vi "Test_SQLQueryVIM1DI64_WorksNoError.vi"(8 "error in (no error)":errorcluster, 11 "TestCase in":refnum<class "Test mysql.lvclass">) -> (0 "error out":errorcluster, 3 "TestCase out":refnum<class "Test mysql.lvclass">)   [LabVIEW 2020, in "DataBase_mysql_Tests.lvlib" / "Test mysql.lvclass"]
uses:
  Test mysql.lvclass
  98ffd0c8-4361-48ce-8721-6d705661544a.vi
  98ffd0c8-4361-48ce-8721-6d705661544a.vi/2b921c3d-a080-433c-a702-8a31cd1244f2.vi
  98ffd0c8-4361-48ce-8721-6d705661544a.vi/7350d3e2-eed7-4e35-bdb1-e124b5b41b91.vi
  <vilib>/Utility/error.llb/Error Cluster From Error Code.vi
  externals/mysql/Source/mysql.net/mysql.lvclass
  <vilib>/addons/_JKI Toolkits/VI Tester/TestCase.llb/TestCase.lvclass
  C:/Program Files/National Instruments/LabVIEW 2020/vi.lib/addons/_JKI Toolkits/VI Tester/TestCase.llb/TestCase.lvclass
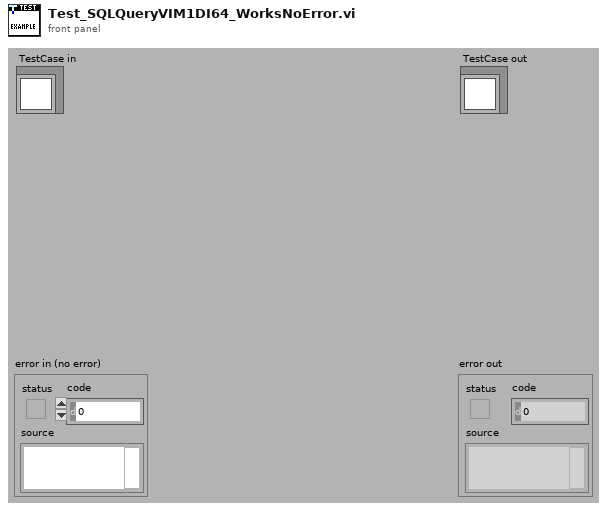
[diagram p1: front panel]
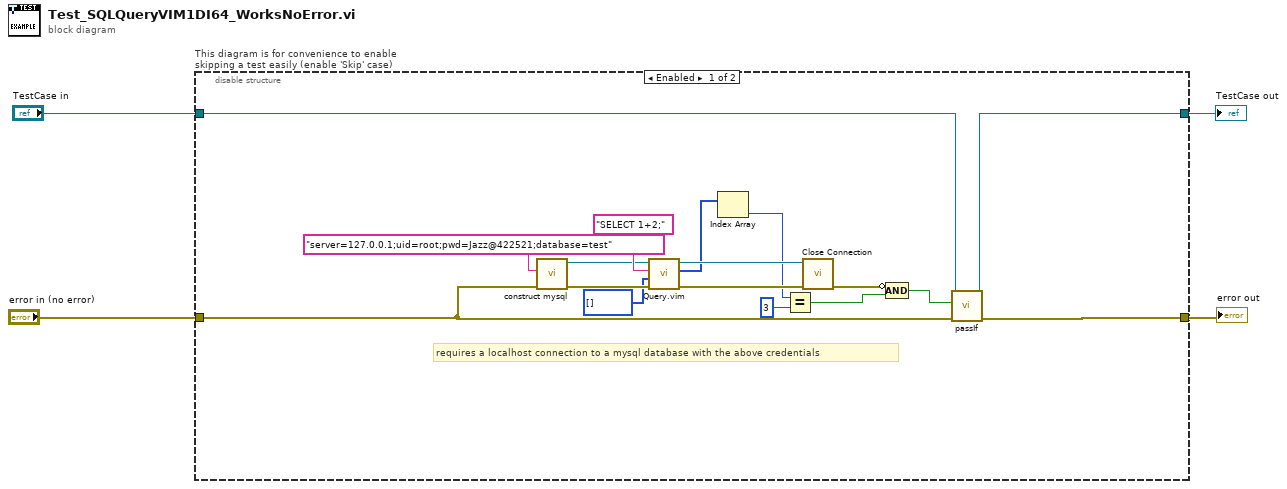
[diagram p0: block diagram]
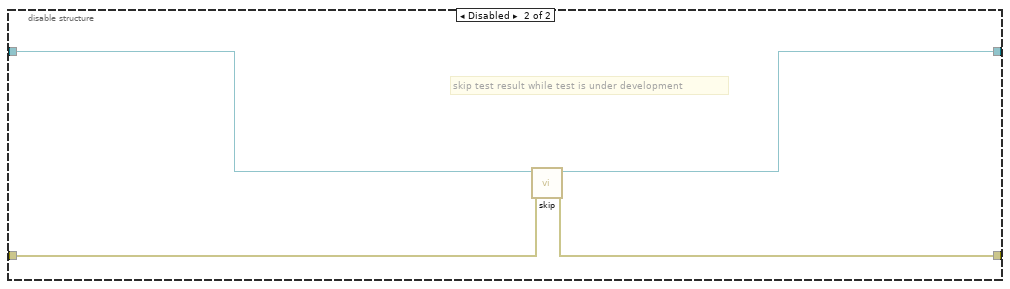
[diagram p2: hidden frame]
diagram:
  n1 = disable-structure "This diagram is for convenience to enable skipping a test easily (enable 'Skip' case)" shown="Enabled" {
    disable-tunnel: "TestCase in" -> [w21 w25]
    disable-tunnel: [w20 w23] -> w1
    disable-tunnel: [w19 w24] -> w3
    disable-tunnel: "error in (no error)" -> [w17 w22]
    frame Enabled {
      # "requires a localhost connection to a mysql database with the above credentials"
      n2 = call "construct mysql.vi"("error in (no error)"=w17, "Connection string"="server=127.0.0.1;uid=root;pwd=Jazz@422521;database=test") -> ("error out"=w11:errorcluster, "mysql out"=w5:refnum<class "mysql.lvclass">)  [unwired: 8 in]
      n3 = call "Query.vim"("error in (no error)"=w11, "Type and Default"=i64[] [], "Query string"="SELECT 1+2;", "IDatabase in"=w5) -> ("error out"=w10:errorcluster, "Result"=w8:i64[], "IDatabase out"=w12:refnum<class "mysql.lvclass">)  [unwired: 5 in]
      n4 = Index Array(array=w8) -> (element=w6:i64)  [unwired: 1 in]
      n5 = Equal?(x=w6, y=i64 3) -> (x = y?=w13:bool)
      n6 = call-dynamic "Close Connection.vi"("error in (no error)"=w10, "mysql in"=w12) -> ("error out"=w16:errorcluster)  [unwired: 8 in, 1 out]
      n7 = Compound Arithmetic op=AND(invert w16, w13) -> (w15:bool)
      n8 = call-dynamic "passIf.vi"("error in (no error)"=w17, "pass"=w15, "TestCase in"=w21) -> ("error out"=w19:errorcluster, "TestCase out"=w20:refnum<class "Test mysql.lvclass">)  [unwired: 7 in]
    }
    frame Disabled {
      # "skip test result while test is under development"
      n9 = call <vilib>:"skip.vi"("error in (no error)"=w22, "TestCase in"=w25) -> ("error out"=w24:errorcluster, "TestCase out"=w23:refnum<class "Test mysql.lvclass">)  [unwired: 8 in]
    }
  }
  "error out" <- w3
  "TestCase out" <- w1
